vi "demo - pico adc finite.vi"() -> ()   [LabVIEW 2024]
doc: "#vi_description \nPlot a ADC data onto a waveform chart until the user presses stop or an error has occurred.\nThetic Engineering Ltd."
uses:
  <instrlib>/HandsOnPi2040/Public/AnaIns.ctl
  <instrlib>/HandsOnPi2040/HandsOnPi2040.lvlib
panel:
  in  "Number of points to acquire":u32=100
  in  "Stop":bool
  out "Waveform Graph":u16[](graph)
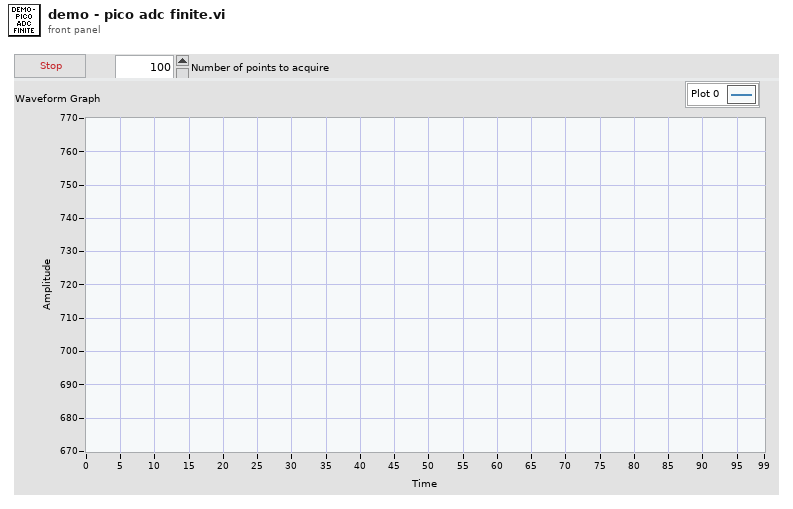
[diagram p1: front panel]
types:
  T1 = typedef "HandsOnPi2040.lvlib/AnaIns.ctl" = enum16{"No AI - Error", "AI1", "AI2"}
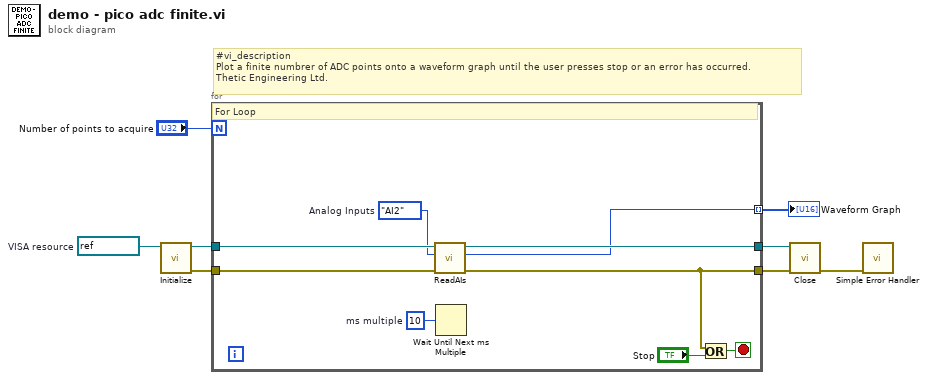
[diagram p0: block diagram]
diagram:
  w4 = refnum<visa-resource-name> "COM3"  # VISA resource
  # "#vi_description \nPlot a finite numbrer of ADC points onto a waveform graph until the user presses stop or an error has occurred.\nThetic Engineering Ltd."
  n1 = call <instrlib>:"Initialize.vi"("VISA resource name"=w4) -> ("error out"=w7:errorcluster, "VISA resource name out"=w8:refnum<visa-resource-name>)  [unwired: 8 in, 1 out]
  n2 = for {
    N: "Number of points to acquire" -> [_]
    tunnel: w8 -> [w15]
    tunnel: w7 -> [w14]
    tunnel: [w13] -> w6
    tunnel: [w11] -> w5
    tunnel: [w9] -> w1 mode=indexing
    stop <- w10 stop-if-true
    w12 = AnaIns."AI2"  # Analog Inputs
    w16 = u32 10  # ms multiple
    # "For Loop"
    n3 = call <instrlib>:"ReadAIs.vi"("error in (no error)"=w14, "Analog Inputs"=w12, "VISA resource name"=w15) -> ("error out"=w11:errorcluster, "Value"=w9:u16, "VISA resource name out"=w13:refnum<visa-resource-name>)  [unwired: 6 in]
    n4 = Wait Until Next ms Multiple(millisecond multiple=w16) -> ()  [unwired: 1 out]
    n5 = Or(x=w11, y="Stop") -> (x .or. y?=w10:bool)
  }
  "Waveform Graph" <- w1
  n6 = call <instrlib>:"Close.vi"("error in (no error)"=w5, "VISA resource name"=w6) -> ("error out"=w3:errorcluster)  [unwired: 9 in]
  n7 = call <vilib>:"Simple Error Handler.vi"("error in (no error)"=w3) -> ()  [unwired: 4 in, 5 out]
